vi "Point in Polygon.vi"   [LabVIEW 2017, in "NI_AAL_Geometry.lvlib"]
doc: "Verifies whether a point is inside a polygon."
uses:
  <vilib>/Analysis/NI_AAL_Geometry.lvlib
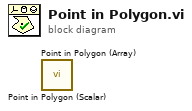
[diagram p0: block diagram]
diagram:
  n1 = call <vilib>:"Point in Polygon (Scalar).vi"() -> ()  [unwired: 10 in, 2 out]
  n2 = call <vilib>:"Point in Polygon (Array).vi"() -> ()  [unwired: 10 in, 2 out]
